vi "Measure_PSF.vi"(8 "error in (no error)":errorcluster, 11 "Signal Channel":enum16{"Red", "Green"}(ring)) -> (0 "error out":errorcluster)   [LabVIEW 2020]
doc: "Use this template to create a dialog box with event handling."
uses:
  Typedefs/Top level VI states.ctl
  Global Variables/gl_Images.vi
panel:
  in  "Delay":u32=1000
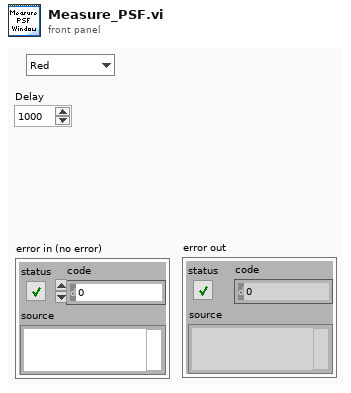
[diagram p1: front panel]
types:
  T1 = typedef "Top level VI states.ctl" = enum16{"None", "Initialise UI", "<STACK PROTOCOL STATES>", "AOL Zstack-START", "AOL Zstack-STOP", "Motor Zstack-START", "Motor Zstack-STOP", "<ACQUISITION PROTOCOL STATES> ", "Functional Acquisition-START", "Functional Acquisition-STOP", "Single Plane Acquisition-START", "Single Plane Acquisition-STOP", "Volume Acquisition-START", "Volume Acquisition-STOP", "<LIVE IMAGING PROTOCOL STATES>", "Live Imaging-START", "Live Imaging-STOP", "Live Plane Imaging-START", "Live Plane Imaging-STOP", "Live Volume Imaging-START", "Live Volume Imaging-STOP", "<MOVEMENT CORRECTION PROTOCOL STATES>", "EXIT"}
  T2 = typedef "IMAQ Image.ctl" = refnum<image>
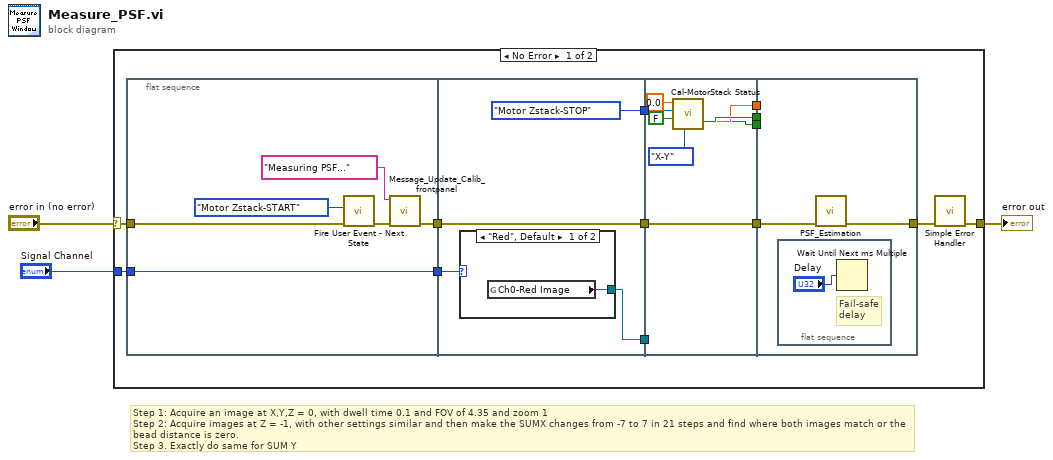
[diagram p0: block diagram]
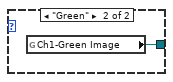
[diagram p2: hidden frame]
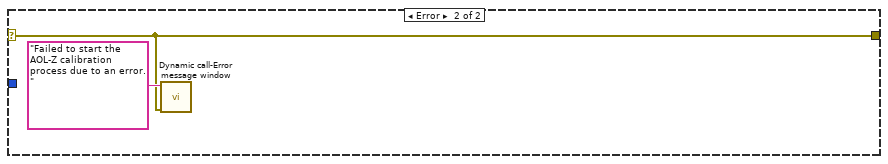
[diagram p3: hidden frame]
diagram:
  # "Step 1: Acquire an image at X,Y,Z = 0, with dwell time 0.1 and FOV of 4.35 and zoom 1\nStep 2: Acquire images at Z = -1, with other settings similar and then make the SUMX changes from -7 to 7 in 21 steps and find where both images match or the bead distance is zero.\nStep 3. Exactly do same for SUM Y"
  n1 = case shown="No Error" "error in (no error)" {
    selector: "error in (no error)" -> [w14 w40]
    tunnel: [w16 w40] -> w3
    tunnel: "Signal Channel" -> [w15 _]
    frame No Error {
      n2 = flat-sequence {
        tunnel: [w21] -> w13
        tunnel: [w17] -> w12
        tunnel: w15 -> [w17]
        tunnel: w14 -> [w22]
        tunnel: [w26] -> w11
        tunnel: w13 -> [w26]
        tunnel: w12 -> [w24]
        tunnel: [w25] -> w10
        tunnel: [Top_level_VI_states."Motor Zstack-STOP" ("Last State")] -> w9
        tunnel: w11 -> [w32]
        tunnel: w10 -> [_]
        tunnel: w9 -> [w36]
        tunnel: [w35] -> w8
        tunnel: [w34] -> w7
        tunnel: [w33] -> w6
        tunnel: [w32] -> w5
        tunnel: w8 -> [_]
        tunnel: w7 -> [_]
        tunnel: w6 -> [_]
        tunnel: w5 -> [w37]
        tunnel: [w38] -> w4
        frame #0 {
          n3 = call "Fire User Event - Next State.vi"("Error In"=w22, "\"UI Handler loop\" case to execute"=Top_level_VI_states."Motor Zstack-START" ("\"UI Handler loop\" case to execute")) -> ("Error Out"=w20:errorcluster)  [unwired: 9 in]
          n4 = call "Message_Update_Calib_frontpanel.vi"("error in (no error)"=w20, "Message"="Measuring PSF...") -> ("error out"=w21:errorcluster)  [unwired: 9 in]
        }
        frame #1 {
          n5 = case shown="\"Red\", Default" w24 {
            tunnel: [w27 w28] -> w25
            frame "Red", Default {
              n6 = global read "gl_Images.vi" "Ch0-Red Image"() -> (w27:T2)
            }
            frame "Green" {
              n7 = global read "gl_Images.vi" "Ch1-Green Image"() -> (w28:T2)
            }
          }
        }
        frame #2 {
          n8 = call "Cal-MotorStack Status.vi"("StageSelection"=enum16{"X-Y", "Z"}."X-Y", "Timed out while waiting for acknowledgement in"=FALSE, "Last State"=w36, "Initial motor position (um)"=sgl 0.0) -> ("Motor timed out or errored out"=w35:bool, "Cancelled"=w33:bool, "Measured cal value"=w34:sgl)  [unwired: 5 in]
        }
        frame #3 {
          n9 = flat-sequence {
            frame #0 {
              # "Fail-safe delay"
              n10 = Wait Until Next ms Multiple(millisecond multiple="Delay") -> ()  [unwired: 1 out]
            }
          }
          n11 = call "PSF_Estimation.vi"("error in (no error)"=w37) -> ("error out"=w38:errorcluster)  [unwired: 10 in]
        }
      }
      n12 = call <vilib>:"Simple Error Handler.vi"("error in (no error)"=w4) -> ("error out"=w16:errorcluster)  [unwired: 4 in, 4 out]
    }
    frame Error {
      n13 = call "Dynamic call-Error message window.vi"("error in (no error)"=w40, "Error Message"="Failed to start the AOL-Z calibration process due to an error.") -> ()  [unwired: 9 in, 1 out]
    }
  }
  "error out" <- w3
